vi "Name To Rename lvlib File Path.vi"(8 "Type":T1, 9 "Rename":string, 10 "Name Library File Path":path) -> (2 "Rename Library File Path":path)   [LabVIEW 2020, in "_Rename.lvlib" / "_Rename.lvclass"]
uses:
  _Rename.lvclass
  _Shared/Type.ctl
  _Shared/_Shared.lvlib
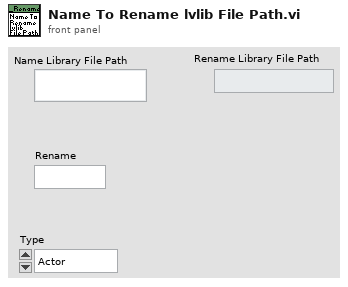
[diagram p1: front panel]
types:
  T1 = typedef "_Shared.lvlib/Type.ctl" = enum16{"Actor", "Msg"}
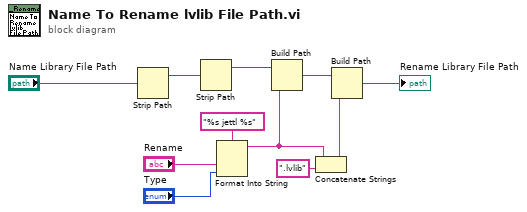
[diagram p0: block diagram]
diagram:
  n1 = Strip Path(path="Name Library File Path") -> (stripped path=w10:path)  [unwired: 1 out]
  n2 = Strip Path(path=w10) -> (stripped path=w9:path)  [unwired: 1 out]
  n3 = Format Into String(format string="%s jettl %s", "Rename", "Type") -> (resulting string=w3:string)  [unwired: 2 in, 1 out]
  n4 = Build Path(base path=w9, name or relative path=w3) -> (appended path=w7:path)
  n5 = Concatenate Strings(w3, ".lvlib" ("string")) -> (w6:string)
  n6 = Build Path(base path=w7, name or relative path=w6) -> (appended path=→"Rename Library File Path":path)
